vi "Flatten Test Parameters.vi"(4 "error in (no error)":errorcluster, 6 "Flattened Test Parameters (\"\")":string, 7 "Test Version":T1 {"Build Date/Time" format="%<%X\n%x>T"}) -> (0 "error out":errorcluster, 3 "Flattened Test Parameters with Version":string)   [LabVIEW 2011]
uses:
  SI.LIB/OGAB Version.ctl
  Flat Report Parameters Cluster.ctl
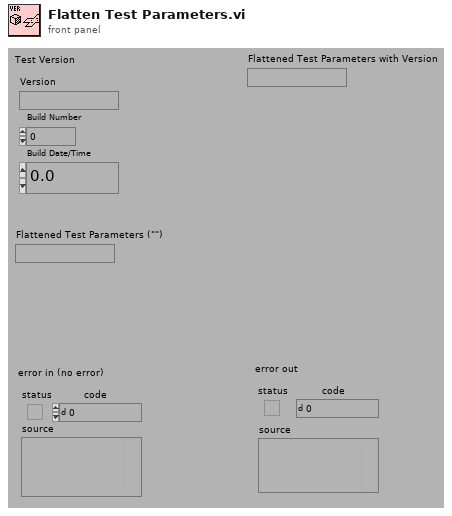
[diagram p1: front panel]
types:
  T1 = typedef "OGAB Version.ctl" = cluster{"Version":string, "Build Number":u32, "Build Date/Time":dbl}
  T2 = typedef "Flat Report Parameters Cluster.ctl" = cluster{"Flattened Test Version":string, "Flattened Test Parameters":string}
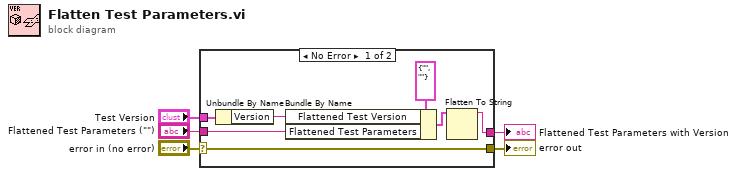
[diagram p0: block diagram]
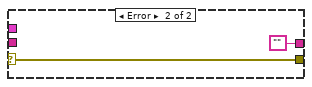
[diagram p2: hidden frame]
diagram:
  n1 = case shown="No Error" "error in (no error)" {
    selector: "error in (no error)" -> [w10 w14]
    tunnel: [w10 w14] -> w4
    tunnel: "Flattened Test Parameters (\"\")" -> [w9 _]
    tunnel: "Test Version" -> [w8 _]
    tunnel: [w6 ""] -> w1
    frame No Error {
      n2 = Unbundle By Name(w8) -> ("Version"=w12:string)
      n3 = Bundle By Name(cluster=T2 {"Flattened Test Version"="", "Flattened Test Parameters"=""} ("Test Report Parameters"), "Flattened Test Version"=w12, "Flattened Test Parameters"=w9) -> (w11:T2)
      n4 = Flatten To String(anything=w11) -> (data string=w6:string)  [unwired: 1 in, 4 out]
    }
    frame Error {
    }
  }
  "error out" <- w4
  "Flattened Test Parameters with Version" <- w1
